vi "ap wireless streaming status t str.vi"(11 "streaming_status":u32(ring) items=["APDM_AP_RECEIVING_UNKNOWN", "APDM_AP_RECEIVING_FROM_ALL_MONITORS", "APDM_AP_RECEIVING_FROM_ALL_MONITORS_AND_CATCHING_UP", "APDM_AP_RECEIVING_FROM_ALL_MONITORS_AND_FALLING_BEHIND", "APDM_AP_NOT_RECEIVING_DATA_FROM_SOME_MONITORS", "APDM_AP_NOT_RECEIVING_DATA_FROM_ANY_MONITORS"]) -> (3 "function return":string)   [LabVIEW 2019, in "apdm.lvlib"]
doc: "APDM_EXPORT const char* apdm_ap_wireless_streaming_status_t_str(const apdm_ap_wireless_streaming_status_t streaming_status);"
uses:
  apdm.lvlib
  Lee Lab/CP FES Walking 2018/Code/Working/LabVIEW/apdm.dll
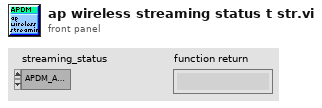
[diagram p1: front panel]
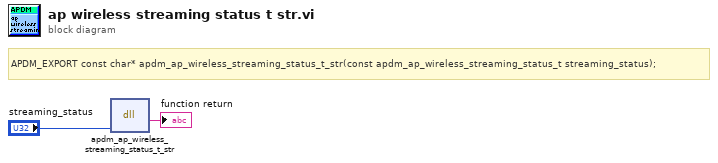
[diagram p0: block diagram]
diagram:
  # "APDM_EXPORT const char* apdm_ap_wireless_streaming_status_t_str(const apdm_ap_wireless_streaming_status_t streaming_status);"
  n1 = dll-call lib="C:/Users/jfalesi/Dropbox/Lee Lab/CP FES Walking 2018/Code/Working/LabVIEW/apdm.*" fn="apdm_ap_wireless_streaming_status_t_str"("streaming_status"="streaming_status") -> (→"function return":string)  [unwired: 4 in, 2 out]
